vi "comms_preprocess_upload_data.vi"(11 "Binary Input Data":string) -> (3 "Binary Output (string)":string)   [LabVIEW 2018]
panel:
  out "*(type *) &x":u8[](array[numeric]) format="%02x"
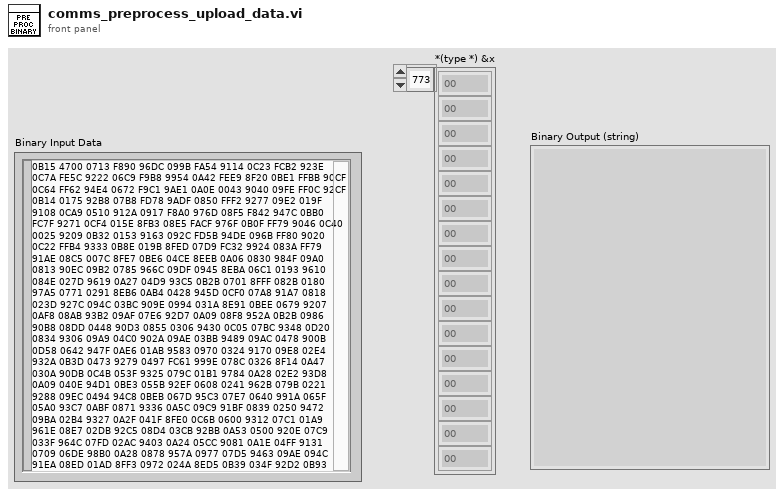
[diagram p1: front panel]
types:
  T1 = enum16{"big-endian, network order", "native, host order", "little-endian"}
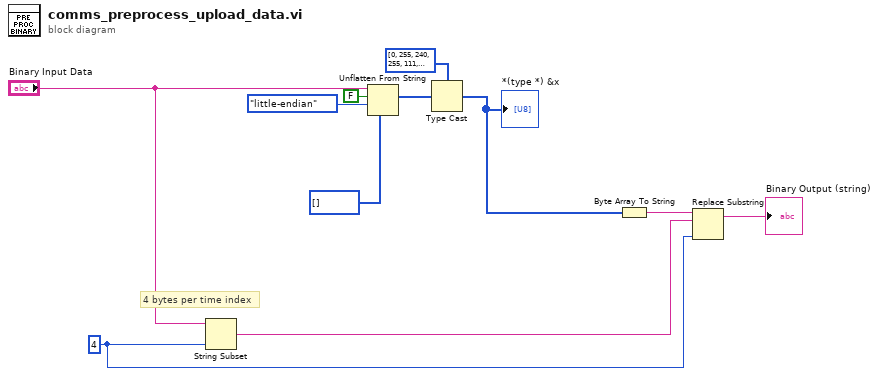
[diagram p0: block diagram]
diagram:
  w1 = 4 ("length (rest)")
  # "4 bytes per time index"
  n1 = String Subset(string="Binary Input Data", length (rest)=w1) -> (substring=w2:string)  [unwired: 1 in]
  n2 = Unflatten From String(type=u16[] [], binary string="Binary Input Data", data includes array or string size? (T)=FALSE, byte order (0:big-endian, network order)=T1."little-endian") -> (value=w6:u16[])  [unwired: 1 in, 2 out]
  n3 = Type Cast(type=u8[] [0, 255, 240, 255, 111, 255, 209, 0, 29, 255, 134, 255, 207, 0, 6, 255, 154, 255, 202, 255, 250, 255, 179, 255, 220, 0, 7, 255, 136, 255, 203, 0, 8, 255, 146, 255, 197, 255, 248, 255, 125, 255, 200, 255, 226, 255, 191, 255, 205, 255, 252, 255, 143, 255, 210, 0, 1, 255, 105, 255, 203, 0, 24, 255, 142, 255, 191, 0, 0, 255, 223, 255, 212, 0, 19, 255, 145, 255, 197, 255, 245, 255, 184, 255, 217, 0, 8, 255, 191, 255, 198, 0, 4, 255, 171, 255, 211, 255, 249, 255, 159, 255, 222, 255, 234, 255, 190, 255, 226, 255, 248, 255, 144, 255, 210, 255, 231, 255, 219, 255, 231, 0, 17, 255, 165, 255, 238, 255, 254, 255, 102, 255, 245, 255, 239, 255, 137, 255, 237, 255, 241, 255, 157, 255, 229, 255, 241, 255, 139, 255, 223, 255, 244, 255, 108, 255, 213, 0, 63, 255, 185, 255, 227, 255, 227, 255, 93, 255, 234, 255, 243, 255, 128, 255, 220, 255, 255, 255, 168, 255, 235, 255, 250, 255, 131, 255, 242, 255, 254, 255, 151, 255, 239, 255, 250, 255, 161, 255, 195, 0, 42, 255, 160, 255, 207, 0, 3, 255, 182, 255, 187, 0, 13, 255, 163, 255, 202, 0, 15, 255, 111, 255, 198, 255, 231, 255, 181, 255, 179, 0, 14, 255, 138, 255, 184, 255, 246, 255, 172, 255, 193, 255, 241, 255, 118, 255, 208, 255, 253, 255, 158, 255, 193, 255, 250, 255, 165, 255, 199, 0, 11, 255, 156, 255, 203, 255, 250, 255, 137, 255, 210, 0, 2, 255, 166, 255, 202, 0, 23, 255, 140, 255, 203, 0, 25, 255, 235, 255, 205, 0, 5, 255, 148, 255, 230, 0, 9, 255, 137, 255, 218, 0, 14, 255, 162, 255, 225, 255, 247, 255, 195, 255, 246, 255, 253, 255, 99, 255, 227, 0, 15, 255, 177, 255, 221, 0, 4, 255, 139, 255, 236, 0, 43, 255, 182, 255, 236, 255, 249, 255, 147, 255, 222, 255, 237, 255, 185, 255, 221, 255, 234, 255, 156, 255, 229, 0, 8, 255, 167, 255, 247, 255, 245, 255, 161, 255, 238, 0, 13, 255, 140, 255, 236, 255, 250, 255, 173, 255, 224, 255, 242, 255, 189, 255, 241, 0, 4, 255, 139, 255, 195, 255, 215, 255, 168, 255, 191, 255, 249, 255, 210, 255, 198, 0, 6, 255, 137, 255, 208, 0, 1, 255, 144, 255, 202, 0, 1, 255, 140, 255, 200, 0, 8, 255, 124, 255, 199, 0, 10, 255, 194, 255, 203, 0, 25, 255, 120, 255, 223, 255, 247, 255, 145, 255, 186, 0, 5, 255, 252, 255, 192, 255, 254, 255, 180, 255, 207, 0, 14, 255, 173, 255, 199, 0, 15, 255, 101, 255, 205, 0, 3, 255, 168, 255, 177, 0, 31, 255, 177, 255, 218, 255, 247, 255, 137, 255, 229, 0, 8, 255, 139, 255, 223, 255, 241, 255, 123, 255, 253, 255, 248, 255, 173, 255, 239, 255, 216, 255, 133, 255, 235, 255, 239, 255, 108, 255, 239, 0, 26, 255, 181, 255, 246, 255, 243, 255, 195, 255, 244, 0, 28, 255, 174, 255, 218, 255, 246, 255, 145, 255, 227, 0, 5, 255, 196, 255, 241, 0, 22, 255, 172, 255, 234, 255, 254, 255, 137, 255, 217, 0, 5, 255, 139, 255, 219, 0, 28, 255, 121, 255, 220, 255, 250, 255, 179, 255, 233, 255, 238, 255, 197, 255, 200, 0, 2, 255, 159, 255, 193, 0, 30, 255, 167, 255, 209, 255, 213, 255, 208, 255, 194, 255, 246, 255, 127, 255, 213, 255, 241, 255, 155, 255, 194, 0, 9, 255, 190, 255, 210, 255, 238, 255, 212, 255, 203, 255, 249, 255, 185, 255, 195, 255, 250, 255, 165, 255, 217, 255, 248, 255, 187, 255, 194, 255, 250, 255, 251, 255, 189, 0, 19, 255, 128, 255, 212, 0, 14, 255, 145, 255, 195, 0, 23, 255, 130, 255, 196, 255, 201, 255, 204, 255, 214, 0, 14, 255, 160, 255, 230, 255, 232, 255, 110, 255, 245, 0, 10, 255, 180, 255, 237, 255, 234, 255, 178, 255, 222, 255, 227, 255, 163, 255, 246, 255, 225, 255, 146, 255, 240, 0, 8, 255, 143, 255, 233, 0, 38, 255, 173, 255, 254, 0, 4, 255, 150, 255, 218, 255, 247, 255, 144, 255, 225, 255, 248, 255, 145, 0, 9, 255, 248, 255, 218, 255, 243, 255, 253, 255, 150, 255, 218, 255, 255, 255, 185, 255, 234, 255, 239, 255, 155, 255, 234, 255, 251, 255, 141, 255] ("unsigned byte array"), x=w6) -> (*(type *) &x=w5:u8[])
  "*(type *) &x" <- w5
  n4 = Byte Array To String(unsigned byte array=w5) -> (string=w4:string)
  n5 = Replace Substring(2:w1, 4:w2, 5:w4) -> (1:→"Binary Output (string)":string)  [unwired: 1 in, 1 out]
